vi "DSF.Engine.Interface.Transceiver.Destroy.vi"(8 "error in (no error)":errorcluster, 11 "Transceiver Interface in":refnum<class "DSF.Engine.Interface.Transceiver.lvclass">) -> (0 "error out":errorcluster)   [LabVIEW 2017, in "Data Sharing Framework Engine.lvlib" / "DSF.Engine.Interface.Transceiver.lvclass"]
uses:
  DSF.Engine.Interface.Transceiver.lvclass
  C:/github/data-sharing-framework/old/dsf core/Source/Engine/Classes/Interface/DSF.Engine.Interface.lvclass
  DSF.Engine.Interface.lvclass
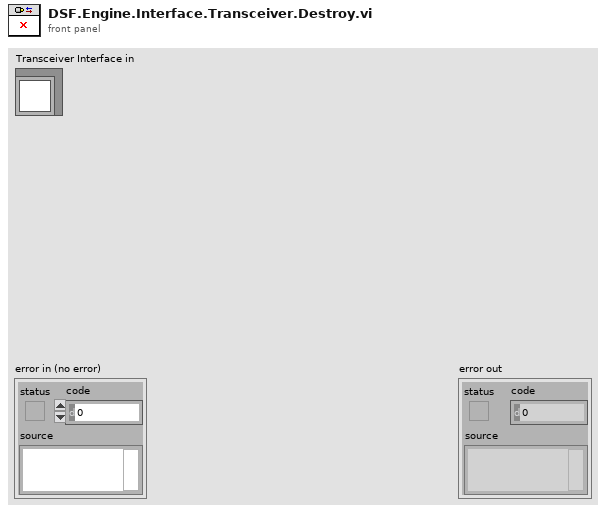
[diagram p1: front panel]
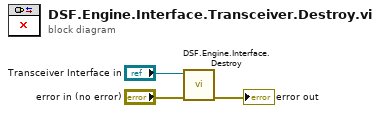
[diagram p0: block diagram]
diagram:
  n1 = call "DSF.Engine.Interface.Destroy.vi"("error in (no error)"="error in (no error)", "Interface in"="Transceiver Interface in") -> ("error out"=→"error out":errorcluster)  [unwired: 7 in, 2 out]
